vi "getPayloadRequirement.vi"(11 "ControlPacket in":refnum<class "ControlPacket.lvclass">) -> (2 "Requirement":T1, 3 "ControlPacket out":refnum<class "ControlPacket.lvclass">)   [LabVIEW 2013, in "ControlPacket.lvclass"]
uses:
  ControlPacket.lvclass
  Requirement -- enum.ctl
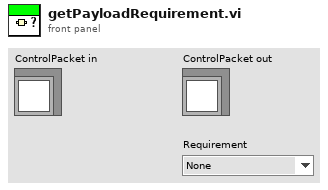
[diagram p1: front panel]
types:
  T1 = typedef "Requirement -- enum.ctl" = enum16{"None", "Optional", "Required"}
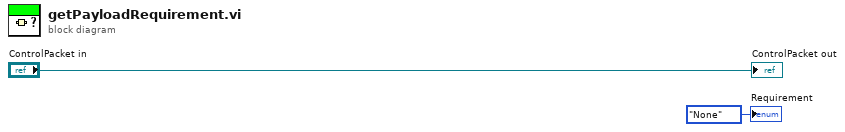
[diagram p0: block diagram]
diagram:
  "ControlPacket out" <- "ControlPacket in"
  "Requirement" <- Requirement_--_enum."None" ("Requirement")
